vi "RMsim_devel02.vi"() -> ()   [LabVIEW 2011]
uses:
  <vilib>/Utility/error.llb/DialogType.ctl
  <vilib>/DAQmx/write.llb/DAQmx Write (Digital Wfm 1Chan NSamp).vi
  <vilib>/DAQmx/write.llb/DAQmx Write (Analog Wfm 1Chan NSamp).vi
  <vilib>/DAQmx/read.llb/DAQmx Read (Analog 1D Wfm NChan NSamp).vi
  <vilib>/DAQmx/create/channels.llb/DAQmx Create Channel (AO-Voltage-Basic).vi
  <vilib>/DAQmx/create/channels.llb/DAQmx Create Channel (AI-Voltage-Basic).vi
  <vilib>/DAQmx/create/channels.llb/DAQmx Create Channel (DO-Digital Output).vi
  <vilib>/DAQmx/configure/timing.llb/DAQmx Timing (Sample Clock).vi
  <vilib>/DAQmx/configure/trigger.llb/DAQmx Start Trigger (Digital Edge).vi
  <vilib>/Waveform/DWDTOps.llb/DWDT Boolean Array to Digital.vi
  <vilib>/Utility/file.llb/Read From Spreadsheet File (DBL).vi
  <vilib>/DAQmx/miscellaneous.llb/DAQmx Fill In Error Info.vi
  <vilib>/Waveform/DWDTOps.llb/DWDT Uncompress Digital.vi
  <vilib>/Utility/file.llb/Write To Spreadsheet File (DBL).vi
panel:
  out "FV gain":dbl[](graph)
  in  "time start":dbl format="%.2f"
  out "Spikes":dbl[][](graph)
  in  "MM Excitation contraction \ndelay (samples)\n(positive only)":dbl=10.0
  in  "burst end (samples)":dbl=1.0 format="%.2f"
  in  "spike frequency (Hz)":dbl=250.0
  in  "MM":bool
  in  "parameters":string="19.751421\r\n0.441873\r\n23.622549\r\n0.916278\r\n0.083826\r\n0.961988\r\n"
  in  "offset":dbl format="%0.2p"
  out "stimulation":dbl[](graph)
  out "Pos from Due (cal/offset)":dbl[](graph)
  out "Force":dbl[][](graph)
  in  "measurement\n   period (s)":dbl=0.5
  in  "wait time before trigger (ms)":u32
  out "AI error":errorcluster
  out "AO error":errorcluster
  out "DO error":errorcluster
  in  "Slope":i32(ring)=10280 items=["Rising"=10280, "Falling"=10171]
  in  "Trigger Source":tag="/Dev1/PFI0"
  out "Analog waveform":waveform(dbl)(graph)
  in  "SAVE?":bool
  out "Last saved":path
  out "Digital Waveform out":digitalwaveform(graph)
  in  "invert digital signal":bool
  in  "data end sound":path=path "C:/WINDOWS/Media/chord.wav"
  out "# samples":i32
  in  "# iterations":i32=1
  in  "Sample Rate":dbl=1000.0 caption="Sample Rate (Hz)" format="%0.2f"
  in  "Physical Channel":tag="Dev1/ai0,Dev1/ai1,Dev1/ai2,Dev1/ai3,Dev1/ai4,Dev1/ai5,Dev1/ai6,Dev1/ai7,Dev1/ai8,Dev1/ai9" caption="Input Physical Channel"
  in  "Minimum Value":dbl=-10.0 format="%0.2f"
  in  "Maximum Value":dbl=10.0 format="%0.2f"
  in  "Physical Channels":tag="Dev1/ao0" caption="Output Physical Channels"
  in  "data start sound":path=path "C:/WINDOWS/Media/chimes.wav"
  in  "Lines":tag="Dev1/port0/line0"
  out "WAITING":bool
  # "PLEASE RENAME THIS FILE BEFORE MODIFYING!"
  # "PLEASE RENAME THIS FILE BEFORE MODIFYING!"
  # "PLEASE RENAME THIS FILE BEFORE MODIFYING!"
  # "ANALOG WAVEFORM"
  # "Activation parameters for RM \n(real muscle --> spikes) or MM \n(muscle model --> active state)"
  # "PLEASE RENAME THIS FILE BEFORE MODIFYING!"
  # "RM"
  # "PLEASE RENAME THIS FILE BEFORE MODIFYING!"
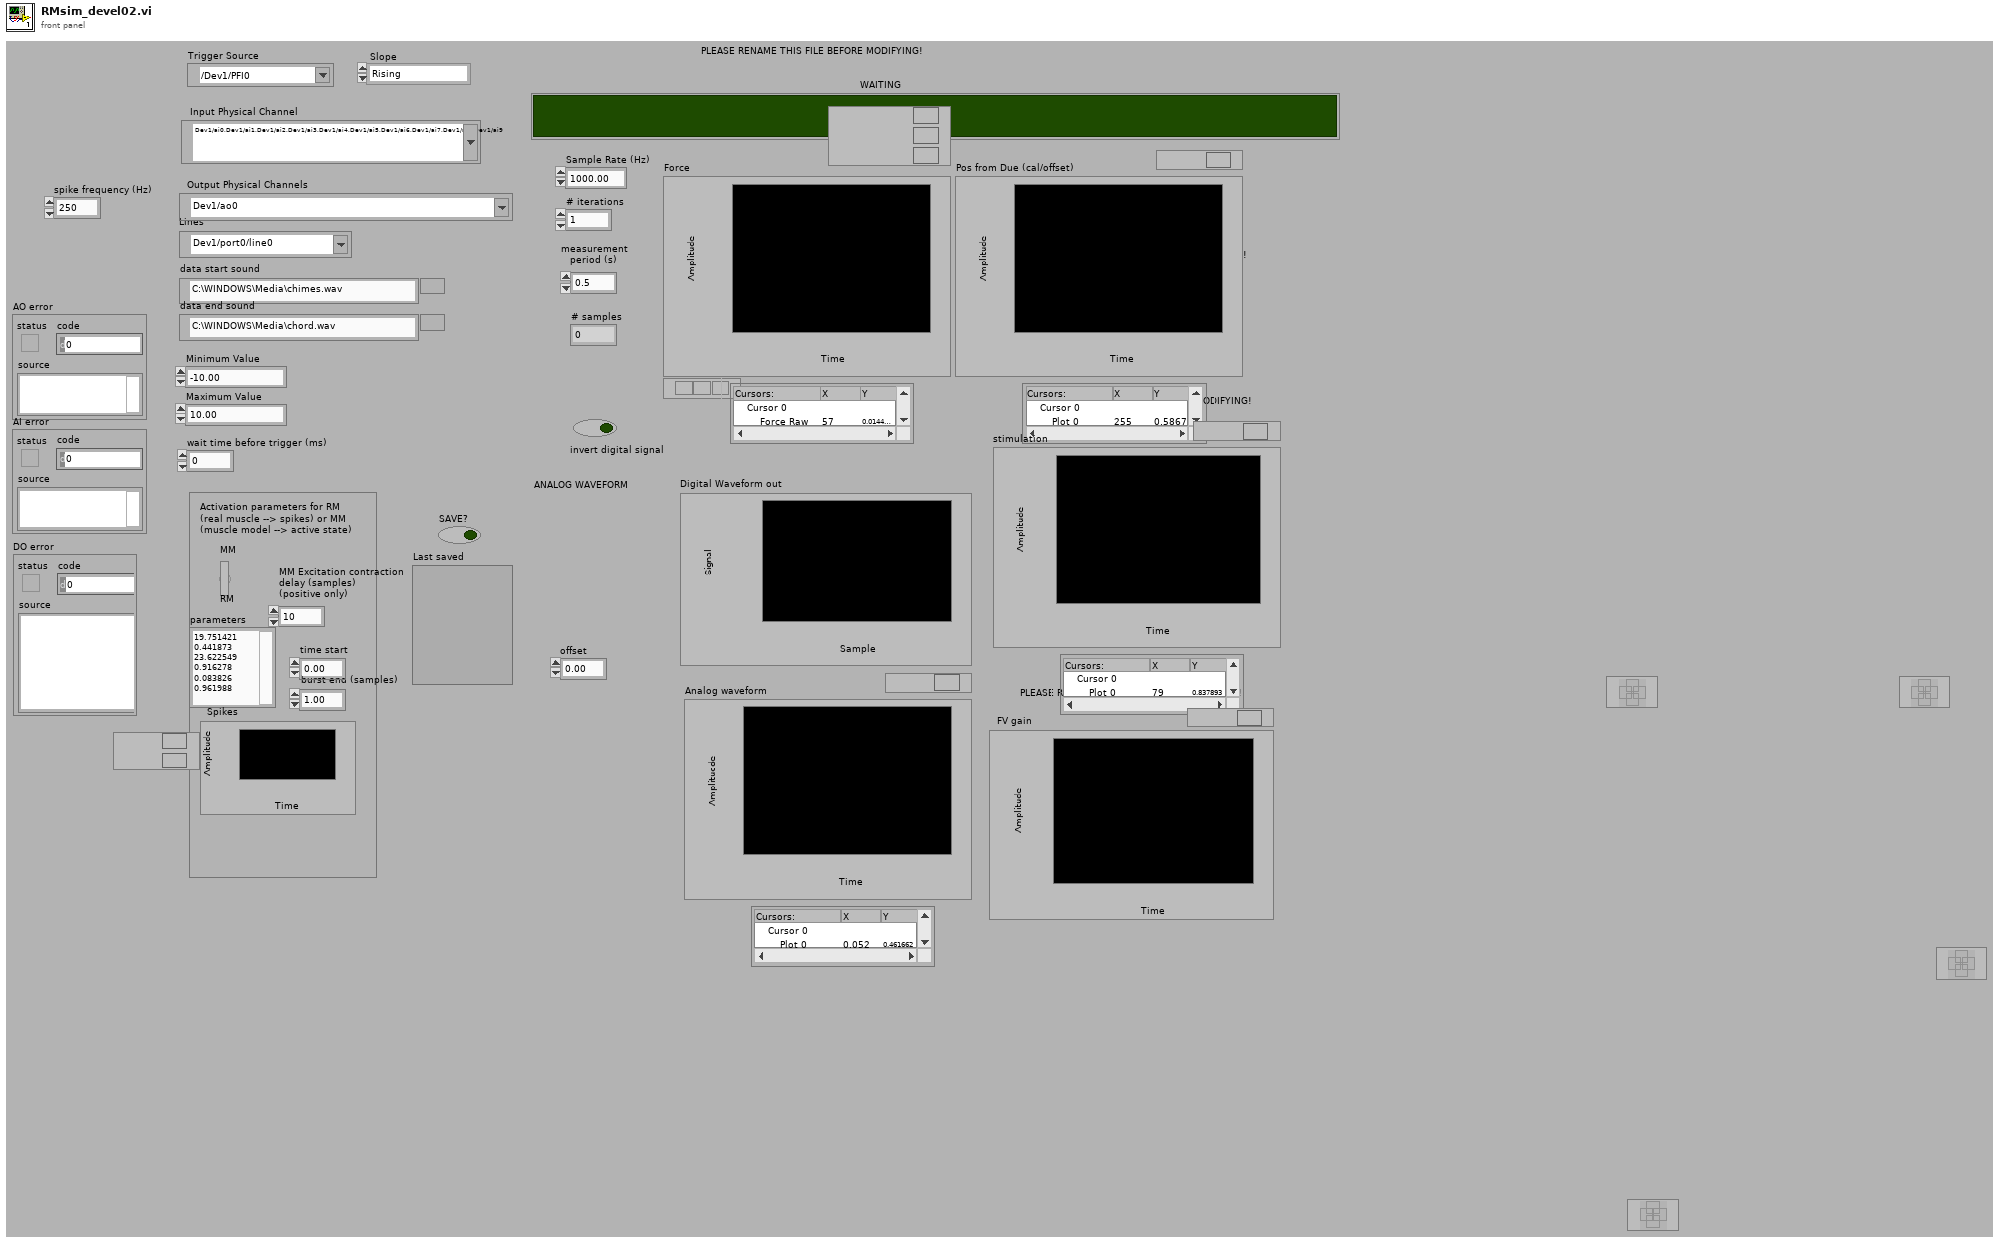
[diagram p1: front panel]
types:
  T1 = typedef "DialogType.ctl" = u16
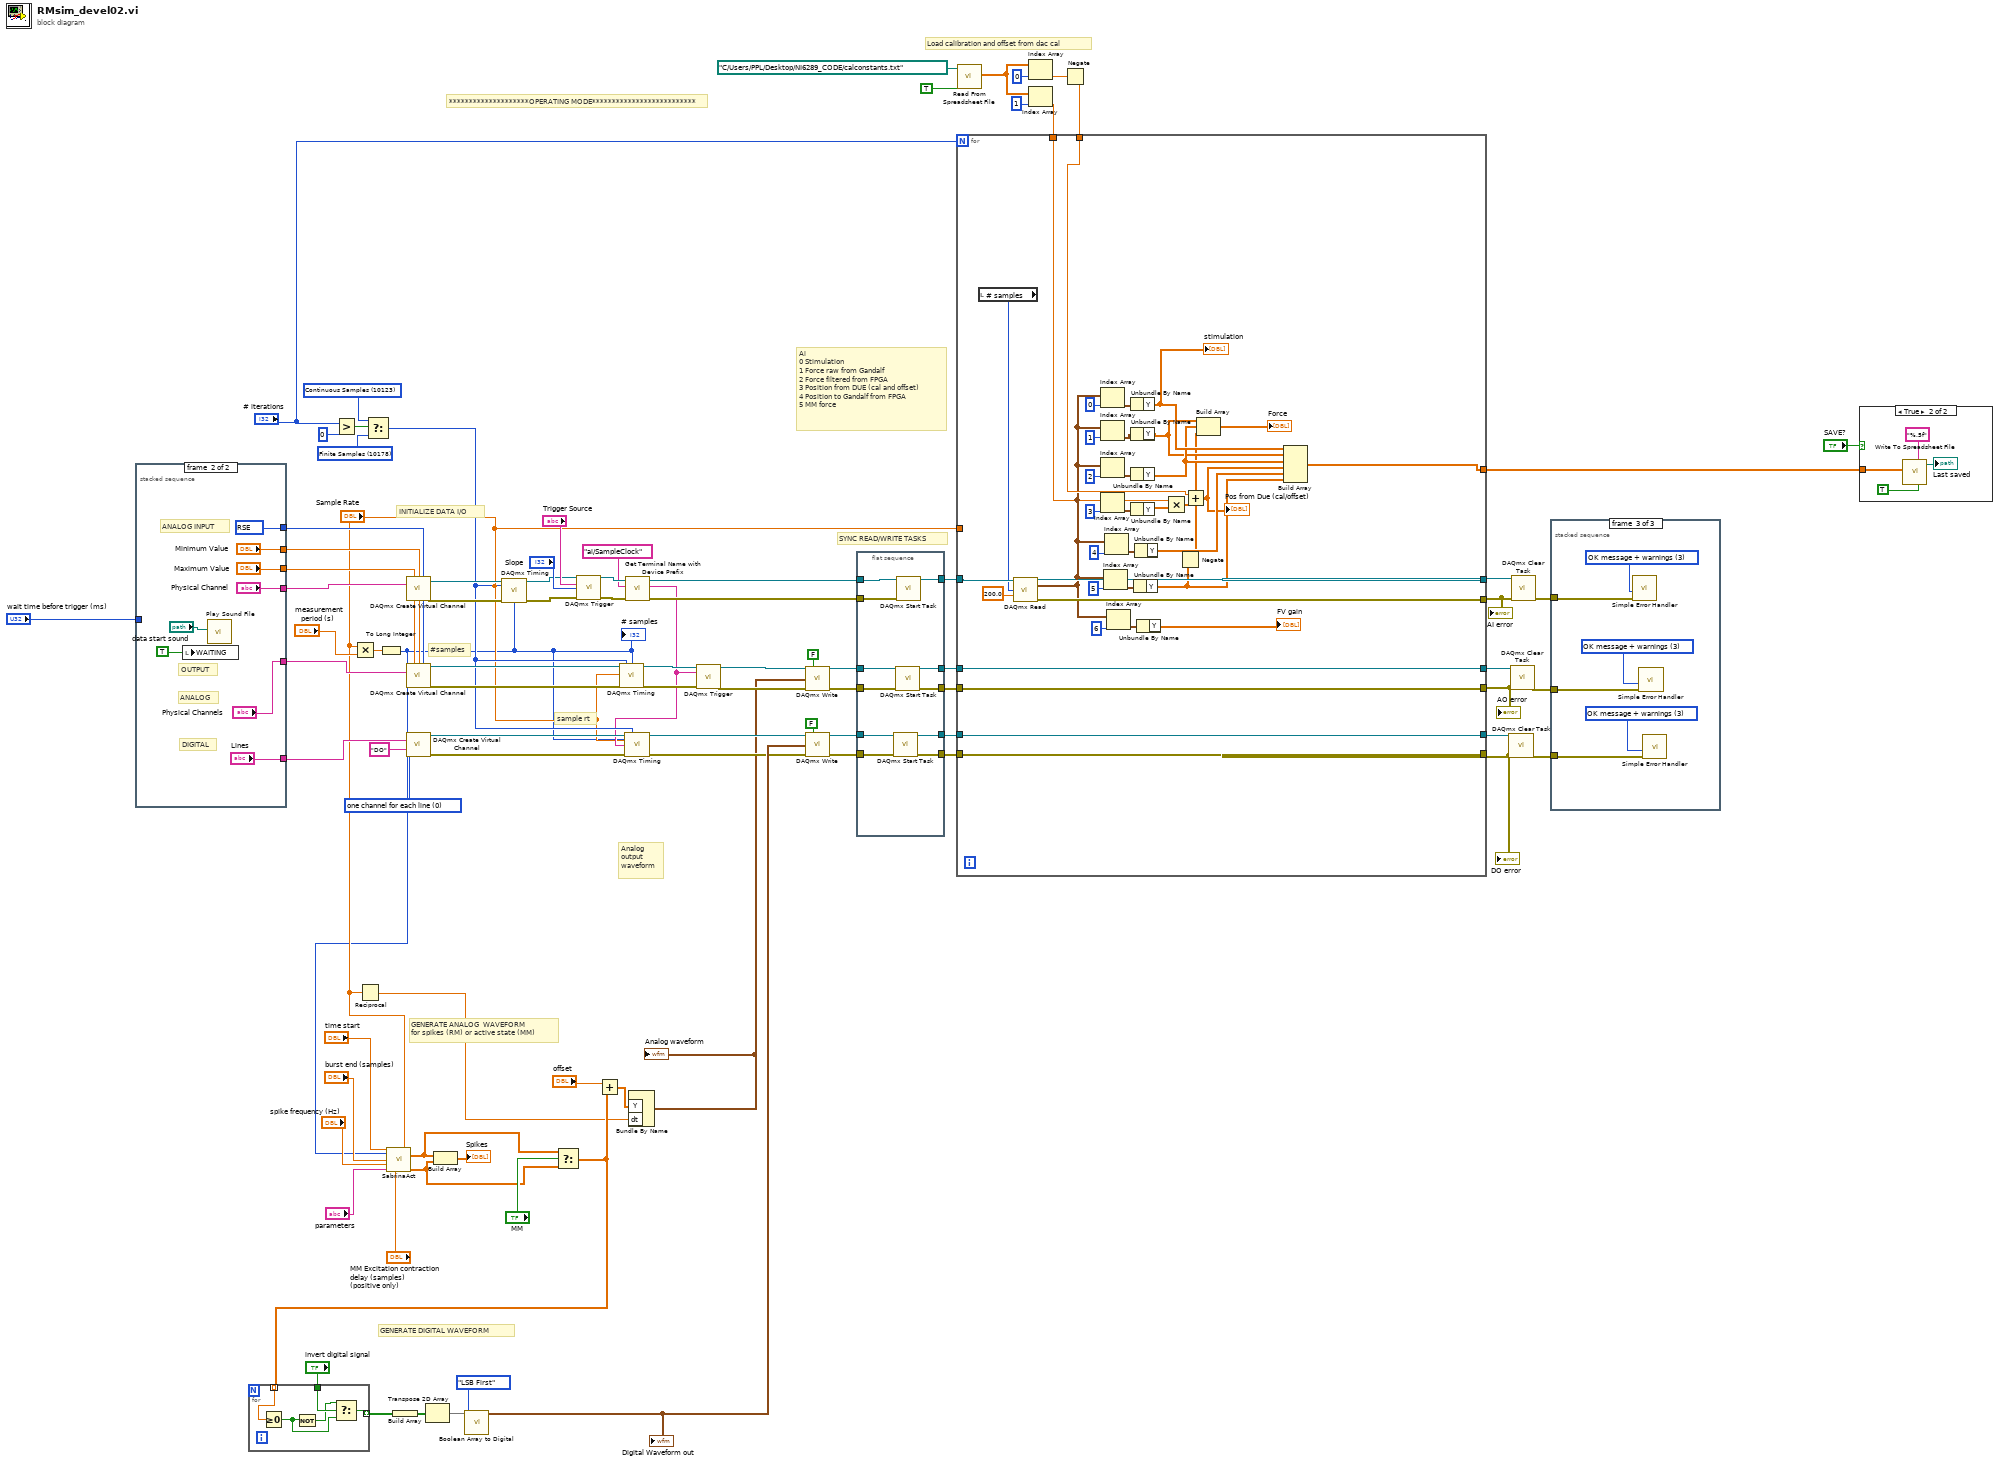
[diagram p0: block diagram]
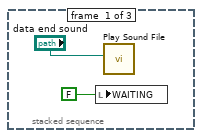
[diagram p2: hidden frame]
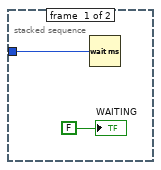
[diagram p5: hidden frame]
diagram:
  w73 = 0 items=["one channel for each line", "one channel for all lines"] ("line grouping")
  w74 = 10178 items=["Finite Samples"=10178, "Continuous Samples"=10123] ("sample mode")
  w76 = 10123 items=["Finite Samples"=10178, "Continuous Samples"=10123] ("sample mode")
  # "Load calibration and offset from dac cal"
  # "Ai\n0 Stimulation\n1 Force raw from Gandalf\n2 Force filtered from FPGA\n3 Position from DUE (cal and offset)\n4 Position to Gandalf from FPGA\n5 MM force"
  # "********************OPERATING MODE**************************"
  # "sample rt"
  # "GENERATE DIGITAL WAVEFORM"
  # "GENERATE ANALOG  WAVEFORM\nfor spikes (RM) or active state (MM)"
  # "Analog\noutput \nwaveform"
  # "SYNC READ/WRITE TASKS"
  # "INITIALIZE DATA I/O"
  # "#samples"
  n1 = stacked-sequence {
    tunnel: [_ "Physical Channel"] -> w90
    tunnel: [_ "Physical Channels"] -> w91
    tunnel: [_ "Minimum Value"] -> w89
    tunnel: [_ "Maximum Value"] -> w88
    tunnel: [_ "Lines"] -> w87
    tunnel: "wait time before trigger (ms)" -> [w93 _]
    tunnel: [_ w95] -> w86
    frame #0 {
      n2 = Wait (ms)(milliseconds to wait=w93) -> ()  [unwired: 1 out]
      "WAITING" <- FALSE ("RECORDING")
    }
    frame #1 {
      w95 = 10083 items=["default"=-1, "RSE"=10083, "NRSE"=10078, "Differential"=10106, "Pseudodifferential"=12529] ("input terminal configuration")
      # "DIGITAL"
      # "ANALOG"
      # "OUTPUT"
      # "ANALOG INPUT"
      n3 = local write "WAITING"(TRUE ("RECORDING")) -> ()
      n4 = call <vilib>:"Play Sound File.vi"("path"="data start sound") -> ()  [unwired: 9 in, 2 out]
    }
  }
  n5 = Greater?(x="# iterations", y=0) -> (0:w75:bool)
  n6 = Multiply(x="Sample Rate", y="measurement\n   period (s)") -> (x*y=w78:dbl)
  n7 = Reciprocal(x="Sample Rate") -> (1/x=w10:dbl)
  n8 = Select(t=w76, s=w75, f=w74) -> (s? t:f=w68:i32)
  n9 = To Long Integer(number=w78) -> (32bit integer=w9:i32)
  "# samples" <- w9
  n10 = call "SabrinaAct.vi"("time start"="time start", "sample rate (Hz)"="Sample Rate", "time end (sampes)"=w9, "burst end (samples)"="burst end (samples)", "spike frequency (Hz)"="spike frequency (Hz)", "parameters"="parameters", "phase delay (samples)"="MM Excitation contraction \ndelay (samples)\n(positive only)") -> ("Activation (1D dbl)"=w14:dbl[], "spikes"=w13:dbl[])  [unwired: 4 in, 3 out]
  n11 = call-poly <vilib>:"DAQmx Create Virtual Channel.vi"("minimum value"=w89, "input terminal configuration"=w86, "physical channels"=w90) -> ("task out"=w81:refnum<k21>, "error out"=w82:errorcluster)  [unwired: 11 in]
  n12 = call-poly <vilib>:"DAQmx Create Virtual Channel.vi"("maximum value"=w88, "minimum value"=w89, "output terminal configuration"=w86, "physical channels"=w91) -> ("task out"=w80:refnum<k21>, "error out"=w79:errorcluster)  [unwired: 10 in]
  n13 = call-poly <vilib>:"DAQmx Create Virtual Channel.vi"("lines"=w87, "name to assign"="DO", "line grouping"=w73) -> ("task out"=w70:refnum<k21>, "error out"=w71:errorcluster)  [unwired: 11 in]
  n14 = Build Array(w14, w13) -> (→"Spikes":dbl[][])
  n15 = call-poly <vilib>:"DAQmx Timing.vi"("task/channels in"=w81, "sample mode"=w68, "samples per channel"=w9, "rate"="Sample Rate", "error in"=w82) -> ("task out"=w34:refnum<k21>, "error out"=w35:errorcluster)  [unwired: 9 in]
  n16 = Select(t=w14, s="MM", f=w13) -> (s? t:f=w12:dbl[])
  n17 = for {
    tunnel: [w106] -> w50 mode=indexing
    tunnel: "invert digital signal" -> [w105]
    tunnel: w12 -> [w104] mode=indexing
    n18 = Greater Or Equal To 0?(x=w104) -> (x >= 0?=w102:bool)
    n19 = Not(x=w102) -> (.not. x?=w103:bool)
    n20 = Select(t=w103, s=w105, f=w102) -> (s? t:f=w106:bool)
  }
  n21 = Build Array(w50) -> (w48:bool[][])
  n22 = Transpose 2D Array(2D array=w48) -> (transposed array=w47:bool[][])
  n23 = call-poly <vilib>:"Boolean Array to Digital.vi"("mode"=enum16{"LSB First", "MSB First"}."LSB First", "boolean array"=w47) -> ("digital waveform"=w45:digitalwaveform)  [unwired: 8 in, 1 out]
  "Digital Waveform out" <- w45
  n24 = call-poly <vilib>:"DAQmx Trigger.vi"("task/channels in"=w34, "source"="Trigger Source", "edge"="Slope", "error in"=w35) -> ("task out"=w37:refnum<k21>, "error out"=w36:errorcluster)  [unwired: 10 in]
  n25 = Add(x="offset", y=w12) -> (x+y=w22:dbl[])
  n26 = call-poly <vilib>:"DAQmx Timing.vi"("task/channels in"=w80, "sample mode"=w68, "samples per channel"=w9, "rate"="Sample Rate", "error in"=w79) -> ("task out"=w33:refnum<k21>, "error out"=w32:errorcluster)  [unwired: 9 in]
  n27 = call "Get Terminal Name with Device Prefix.vi"("error in (no error)"=w36, "Local Terminal Name"="ai/SampleClock", "task/channels in"=w37) -> ("error out"=w41:errorcluster, "Terminal Name with Device Prefix"=w27:tag, "task out"=w42:refnum<k21>)  [unwired: 6 in]
  n28 = call-poly <vilib>:"DAQmx Timing.vi"("task/channels in"=w70, "sample mode"=w68, "samples per channel"=w9, "rate"="Sample Rate", "source"=w27, "error in"=w71) -> ("task out"=w29:refnum<k21>, "error out"=w28:errorcluster)  [unwired: 8 in]
  n29 = Bundle By Name("Y"=w22, "dt"=w10) -> (w24:waveform(dbl))  [unwired: 1 in]
  "Analog waveform" <- w24
  n30 = call-poly <vilib>:"DAQmx Trigger.vi"("task/channels in"=w33, "source"=w27, "error in"=w32) -> ("task out"=w31:refnum<k21>, "error out"=w25:errorcluster)  [unwired: 11 in]
  n31 = call-poly <vilib>:"DAQmx Write.vi"("task/channels in"=w31, "auto start"=FALSE, "data"=w24, "error in"=w25) -> ("task out"=w65:refnum<k21>, "error out"=w43:errorcluster)  [unwired: 9 in, 1 out]
  n32 = call-poly <vilib>:"DAQmx Write.vi"("task/channels in"=w29, "auto start"=FALSE, "data"=w45, "error in"=w28) -> ("task out"=w66:refnum<k21>, "error out"=w44:errorcluster)  [unwired: 9 in, 1 out]
  n33 = flat-sequence {
    tunnel: [w115] -> w60
    tunnel: [w114] -> w59
    tunnel: [w113] -> w56
    tunnel: [w112] -> w55
    tunnel: [w109] -> w40
    tunnel: w66 -> [w117]
    tunnel: w65 -> [w116]
    tunnel: w44 -> [w111]
    tunnel: w43 -> [w110]
    tunnel: w42 -> [w108]
    tunnel: w41 -> [w107]
    frame #0 {
      n34 = call <vilib>:"DAQmx Start Task.vi"("task/channels in"=w117, "error in"=w111) -> ("task out"=w114:refnum<k21>, "error out"=w113:errorcluster)  [unwired: 12 in]
      n35 = call <vilib>:"DAQmx Start Task.vi"("task/channels in"=w116, "error in"=w110) -> ("task out"=w115:refnum<k21>, "error out"=w112:errorcluster)  [unwired: 12 in]
      n36 = call <vilib>:"DAQmx Start Task.vi"("task/channels in"=w108, "error in"=w107) -> ("task out"=w109:refnum<k21>)  [unwired: 12 in, 1 out]
    }
  }
  n37 = call-poly <vilib>:"Read From Spreadsheet File.vi"("transpose (no:F)"=TRUE, "file path (dialog if empty)"=path "C:/Users/PPL/Desktop/NI6289_CODE/calconstants.txt") -> ("first row"=w6:dbl[])  [unwired: 5 in, 4 out]
  n38 = Index Array(array=w6, index=1) -> (element=w2:dbl)
  n39 = Index Array(array=w6, index=0) -> (element=w3:dbl)
  n40 = Negate(x=w3) -> (-x=w1:dbl)
  n41 = for {
    N: "# iterations" -> [_]
    tunnel: [w155] -> w62
    tunnel: [w154] -> w61
    tunnel: w40 -> [w147]
    tunnel: [w145] -> w58
    tunnel: w60 -> [w145]
    tunnel: [w144] -> w57
    tunnel: w59 -> [w144]
    tunnel: [w143] -> w54
    tunnel: w56 -> [w143]
    tunnel: [w142] -> w53
    tunnel: w55 -> [w142]
    tunnel: [w138] -> w83
    tunnel: "Sample Rate" -> [_]
    tunnel: w2 -> [w133]
    tunnel: w1 -> [w130]
    n42 = local read "# samples"() -> (w146:i32)
    n43 = call-poly <vilib>:"DAQmx Read.vi"("task/channels in"=w147, "number of samples per channel"=w146, "timeout"=200.0) -> ("task out"=w155:refnum<k21>, "data"=w119:waveform(dbl)[], "error out"=w154:errorcluster)  [unwired: 10 in]
    n44 = Index Array(array=w119, index=0) -> (element=w153:waveform(dbl))
    n45 = Index Array(array=w119, index=1) -> (element=w150:waveform(dbl))
    n46 = Index Array(array=w119, index=2) -> (element=w149:waveform(dbl))
    n47 = Index Array(array=w119, index=3) -> (element=w140:waveform(dbl))
    n48 = Index Array(array=w119, index=5) -> (element=w124:waveform(dbl))
    n49 = Index Array(array=w119, index=4) -> (element=w135:waveform(dbl))
    n50 = Index Array(array=w119, index=6) -> (element=w120:waveform(dbl))
    n51 = Unbundle By Name(w153) -> ("Y"=w137:dbl[])
    "stimulation" <- w137
    n52 = Unbundle By Name(w150) -> ("Y"=w128:dbl[])
    n53 = Unbundle By Name(w149) -> ("Y"=w129:dbl[])
    n54 = Unbundle By Name(w140) -> ("Y"=w132:dbl[])
    n55 = Unbundle By Name(w124) -> ("Y"=w123:dbl[])
    n56 = Unbundle By Name(w135) -> ("Y"=w134:dbl[])
    n57 = Unbundle By Name(w120) -> ("Y"=→"FV gain":dbl[])
    n58 = Multiply(x=w133, y=w132) -> (x*y=w131:dbl[])
    n59 = Negate(x=w123) -> (-x=w122:dbl[])
    n60 = Add(x=w130, y=w131) -> (x+y=w126:dbl[])
    "Pos from Due (cal/offset)" <- w126
    n61 = Build Array(w128, w129, w122) -> (→"Force":dbl[][])
    n62 = Build Array(w137, w128, w129, w126, w134, w123) -> (w138:dbl[][])
  }
  "DO error" <- w54
  "AO error" <- w53
  "AI error" <- w61
  n63 = call <vilib>:"DAQmx Clear Task.vi"("task in"=w57, "error in"=w54) -> ("error out"=w52:errorcluster)  [unwired: 13 in]
  n64 = call <vilib>:"DAQmx Clear Task.vi"("task in"=w58, "error in"=w53) -> ("error out"=w51:errorcluster)  [unwired: 13 in]
  n65 = call <vilib>:"DAQmx Clear Task.vi"("task in"=w62, "error in"=w61) -> ("error out"=w63:errorcluster)  [unwired: 13 in]
  n66 = stacked-sequence {
    tunnel: w63 -> [_ _ w163]
    tunnel: w52 -> [_ _ w159]
    tunnel: w51 -> [_ _ w158]
    frame #0 {
      n67 = local write "WAITING"(FALSE ("RECORDING")) -> ()
      n68 = call <vilib>:"Play Sound File.vi"("path"="data end sound") -> ()  [unwired: 9 in, 2 out]
    }
    frame #1 {
    }
    frame #2 {
      w161 = T1 3 items=["no dialog", "OK message", "continue or stop message", "OK message + warnings", "continue/stop + warnings"] ("type of dialog (OK msg:1)")
      w160 = T1 3 items=["no dialog", "OK message", "continue or stop message", "OK message + warnings", "continue/stop + warnings"] ("type of dialog (OK msg:1)")
      w162 = T1 3 items=["no dialog", "OK message", "continue or stop message", "OK message + warnings", "continue/stop + warnings"] ("type of dialog (OK msg:1)")
      n69 = call <vilib>:"Simple Error Handler.vi"("type of dialog (OK msg:1)"=w162, "error in (no error)"=w163) -> ()  [unwired: 3 in, 5 out]
      n70 = call <vilib>:"Simple Error Handler.vi"("type of dialog (OK msg:1)"=w160, "error in (no error)"=w158) -> ()  [unwired: 3 in, 5 out]
      n71 = call <vilib>:"Simple Error Handler.vi"("type of dialog (OK msg:1)"=w161, "error in (no error)"=w159) -> ()  [unwired: 3 in, 5 out]
    }
  }
  n72 = case shown="True" "SAVE?" {
    tunnel: w83 -> [_ w165]
    frame False {
    }
    frame True {
      n73 = call-poly <vilib>:"Write To Spreadsheet File.vi"("transpose? (no:F)"=TRUE, "format (%.3f)"="%.5f", "2D data"=w165) -> ("new file path (Not A Path if cancelled)"=→"Last saved":path)  [unwired: 5 in]
    }
  }
